vi "load data-from folder.vi"() -> (0 "cancelled":bool, 3 "selected files":path[](array[path]))   [LabVIEW 2025]
panel:
  in  "wild card":string
  in  "selection":T1(ring)
  in  "Done":bool
  in  "files":cluster{"String":string, "Boolean":bool}[](array[cluster]) caption="Select data files to be imported"
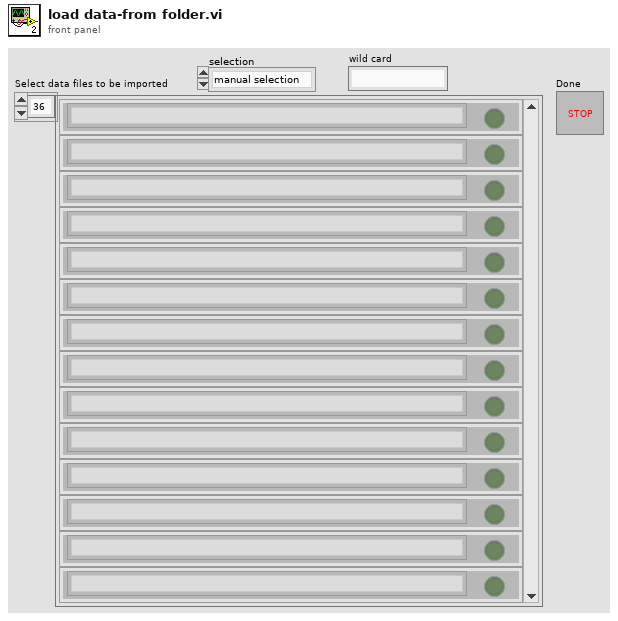
[diagram p1: front panel]
types:
  T1 = enum16{"manual selection", "select all", "unselect all", "inverse selection", "use wild card"}
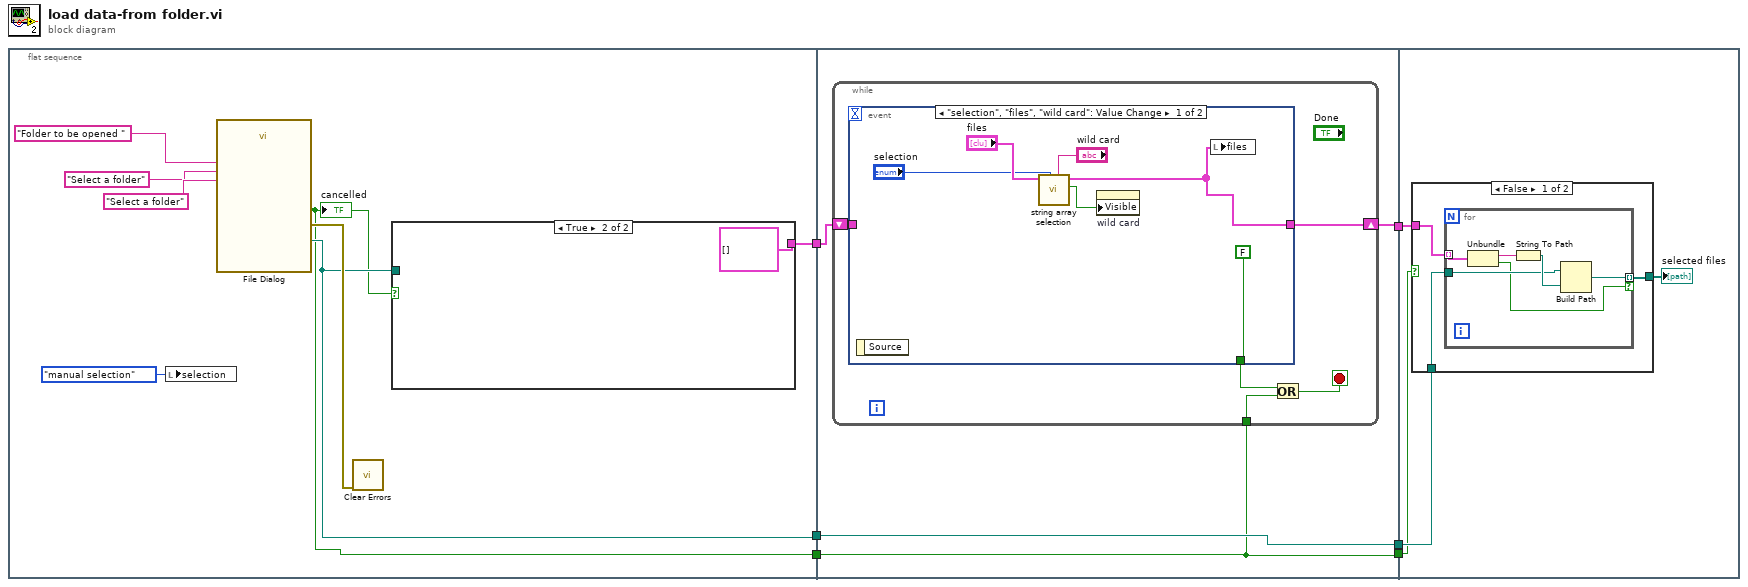
[diagram p0: block diagram]
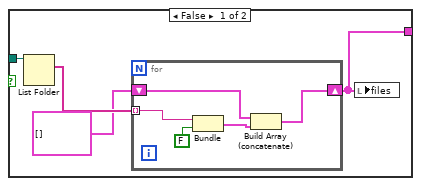
[diagram p2: hidden frame]
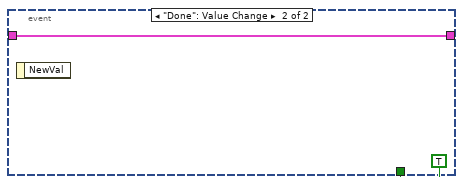
[diagram p3: hidden frame]
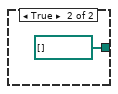
[diagram p4: hidden frame]
diagram:
  n1 = flat-sequence {
    tunnel: [w13] -> w4
    tunnel: [w12] -> w3
    tunnel: [w8] -> w1
    tunnel: [w28] -> w6
    tunnel: [w27] -> w5
    tunnel: w4 -> [w27]
    tunnel: w3 -> [w26]
    tunnel: [w26] -> w2
    tunnel: w1 -> [w25]
    tunnel: w6 -> [w45]
    tunnel: w5 -> [w44]
    tunnel: w2 -> [w42]
    frame #0 {
      n2 = local write "selection"(T1."manual selection" ("selection")) -> ()
      n3 = call "File Dialog"("prompt"="Select a folder", "button label"="Select a folder", "pattern label"="Folder to be opened ") -> ("selected path"=w13:path, "cancelled"=w12:bool, "error out"=w14:errorcluster)  [unwired: 9 in, 1 out]
      "cancelled" <- w12
      n4 = call <vilib>:"Clear Errors.vi"("error in (no error)"=w14) -> ()  [unwired: 5 in, 2 out]
      n5 = case shown="True" w12 {
        tunnel: w13 -> [w16 _]
        tunnel: [w15 cluster{string, bool}[] []] -> w8
        frame False {
          n6 = List Folder(path=w16) -> (filenames=w18:string[])  [unwired: 3 in, 3 out]
          n7 = for {
            tunnel: w18 -> [w22] mode=indexing
            shift-right: [w20] -> w15
            shift-left: cluster{string, bool}[] [] -> [w19]
            n8 = Bundle(w22, FALSE) -> (w21:cluster{string, bool})  [unwired: 1 in]
            n9 = Build Array (concatenate)(w19, w21) -> (w20:cluster{string, bool}[])
          }
          n10 = local write "files"(w15) -> ()
        }
        frame True {
        }
      }
    }
    frame #1 {
      n11 = while {
        tunnel: w26 -> [w32]
        shift-right: [w31] -> w28
        shift-left: w25 -> [w29]
        stop <- w33 stop-if-true
        n12 = event shown="[0] \"selection\", \"files\", \"wild card\": Value Change" {
          selector: _ -> [_ _]
          dyn-events: _ -> [_ _]
          timeout: _ -> [_ _]
          tunnel: [w34 w40] -> w31
          tunnel: [FALSE TRUE] -> w30
          tunnel: w29 -> [_ w40]
          event "selection", "files", "wild card": Value Change {
            n13 = event-data() -> ()  [unwired: 1 in, 1 out]
            n14 = call "string array selection.vi"("regular expression"="wild card", "selection"="selection", "files"="files") -> ("wild card?"=w35:bool, "files 2"=w34:cluster{"String":string, "Boolean":bool}[])  [unwired: 7 in]
            n15 = property on="wild card" class="Str"("Visible"=w35) -> ()  [unwired: 2 in, 2 out]
            n16 = local write "files"(w34) -> ()
          }
          event "Done": Value Change {
            n17 = event-data() -> ()  [unwired: 1 in, 1 out]
          }
        }
        n18 = Or(x=w30, y=w32) -> (x .or. y?=w33:bool)
      }
    }
    frame #2 {
      n19 = case shown="False" w42 {
        tunnel: w45 -> [w48 _]
        tunnel: w44 -> [w47 _]
        tunnel: [w46 path[] []] -> w43
        frame False {
          n20 = for {
            tunnel: w48 -> [w54] mode=indexing
            tunnel: w47 -> [w51]
            tunnel: [w50] -> w46 mode=indexing if=w49
            n21 = Unbundle(w54) -> (w53:string, w49:bool)
            n22 = String To Path(string=w53) -> (path=w52:path)
            n23 = Build Path(base path=w51, name or relative path=w52) -> (appended path=w50:path)
          }
        }
        frame True {
        }
      }
      "selected files" <- w43
    }
  }
